vi "Place.vi"(4 "Side":T1=enum."right", 9 "Part Name":string="Large Gear", 11 "Location":T2={"x"=50.0, "y"=900.0, "a"=900.0, "Name"="Large Gear"}) -> (0 "error out":errorcluster)   [LabVIEW 2013]
uses:
  ROS/Code/SubVIs/BaxterSide.ctl
  Move/Move Reference.vi
  Move/Move XYZA.vi
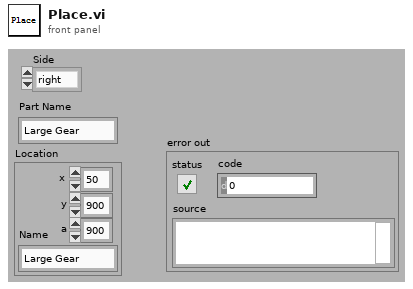
[diagram p1: front panel]
types:
  T1 = typedef "BaxterSide.ctl" = enum16{"left", "right"}
  T2 = cluster{"x":dbl, "y":dbl, "a":dbl, "Name":string}
  T3 = cluster{"X":dbl, "Y":dbl, "Z":dbl, "O":dbl, "A":dbl, "T":dbl}
  T4 = typedef "NI_Matrix.lvlib/RealMatrix.ctl" = dbl[][]
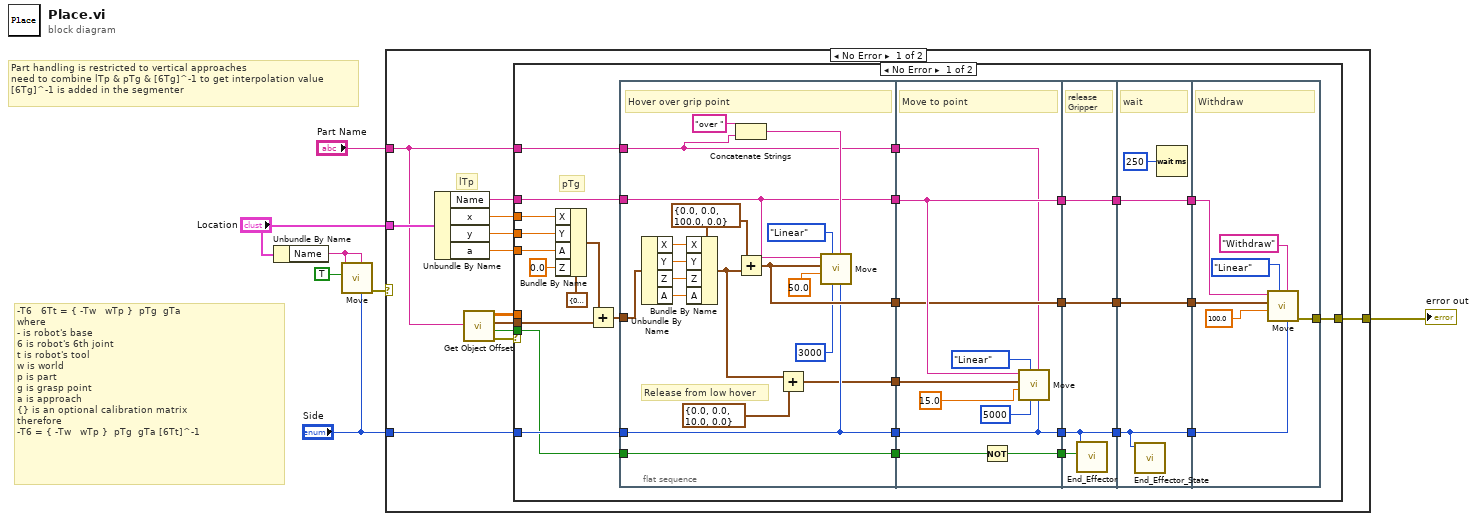
[diagram p0: block diagram]
diagram:
  # "Part handling is restricted to vertical approaches\nneed to combine lTp & pTg & [6Tg]^-1 to get interpolation value\n[6Tg]^-1 is added in the segmenter"
  # "-T6   6Tt = { -Tw   wTp }  pTg  gTa\nwhere \n- is robot's base\n6 is robot's 6th joint\nt is robot's tool\nw is world\np is part\ng is grasp point\na is approach\n{} is an optional calibration matrix\ntherefore\n-T6 = { -Tw   wTp }  pTg  gTa [6Tt]^-1"
  n1 = Unbundle By Name("Location") -> ("Name"=w3:string)
  n2 = call-poly "Move.vi"("Side"="Side", "Label"=w3, "To Reference"=TRUE, "Location"=w3) -> ("error out"=w5:errorcluster)  [unwired: 7 in]
  n3 = case shown="No Error" w5 {
    selector: w5 -> [_ w94]
    tunnel: [w19 w94] -> w7
    tunnel: "Location" -> [w13 _]
    tunnel: "Side" -> [w15 _]
    tunnel: "Part Name" -> [w8 _]
    frame No Error {
      # "lTp"
      n4 = Unbundle By Name(w13) -> ("Name"=w12:string, "x"=w11:dbl, "y"=w10:dbl, "a"=w9:dbl)
      n5 = call "Get Object Offset.vi"("Label"=w8) -> ("error out"=w17:errorcluster, "GraspClose"=w16:bool, "XYZOAT"=w14:T3, "T"=w18:T4)  [unwired: 7 in]
      n6 = case shown="No Error" w17 {
        selector: w17 -> [_ w93]
        tunnel: [w48 w93] -> w19
        tunnel: w18 -> [_ _]
        tunnel: w16 -> [w21 _]
        tunnel: w15 -> [w24 _]
        tunnel: w14 -> [w46 _]
        tunnel: w12 -> [w45 _]
        tunnel: w11 -> [w44 _]
        tunnel: w10 -> [w43 _]
        tunnel: w9 -> [w42 _]
        tunnel: w8 -> [w23 _]
        frame No Error {
          # "pTg"
          n7 = Bundle By Name(cluster=T3 {"X"=0.0, "Y"=0.0, "Z"=0.0, "O"=0.0, "A"=0.0, "T"=0.0} ("XYZOAT"), "X"=w44, "Y"=w43, "A"=w42, "Z"=0.0) -> (w47:T3)
          n8 = Add(x=w47, y=w46) -> (x+y=w40:T3)
          n9 = flat-sequence {
            tunnel: [w53] -> w39
            tunnel: [w55] -> w38
            tunnel: [w51] -> w37
            tunnel: [w57] -> w36
            tunnel: [w56] -> w35
            tunnel: w24 -> [w53]
            tunnel: w21 -> [w55]
            tunnel: w40 -> [w63]
            tunnel: w45 -> [w57]
            tunnel: w23 -> [w52]
            tunnel: [w52] -> w22
            tunnel: w39 -> [w71]
            tunnel: [w71] -> w34
            tunnel: w38 -> [w73]
            tunnel: [w68] -> w33
            tunnel: w37 -> [w75]
            tunnel: w36 -> [w74]
            tunnel: [w74] -> w32
            tunnel: w35 -> [w72]
            tunnel: [w72] -> w31
            tunnel: w22 -> [w69]
            tunnel: w34 -> [w79]
            tunnel: [w79] -> w30
            tunnel: w33 -> [w78]
            tunnel: w32 -> [w81]
            tunnel: [w81] -> w28
            tunnel: w31 -> [w80]
            tunnel: [w80] -> w26
            tunnel: w30 -> [w82]
            tunnel: [w82] -> w29
            tunnel: w28 -> [w85]
            tunnel: [w85] -> w27
            tunnel: w26 -> [w84]
            tunnel: [w84] -> w25
            tunnel: w29 -> [w86]
            tunnel: [w92] -> w48
            tunnel: w27 -> [w87]
            tunnel: w25 -> [w88]
            frame #0 {
              w58 = cluster{"X":dbl, "Y":dbl, "Z":dbl, "A":dbl} {"X"=0.0, "Y"=0.0, "Z"=100.0, "A"=0.0} ("XYZA")
              # "Release from low hover"
              # "Hover over grip point"
              n10 = Unbundle By Name(w63) -> ("X"=w62:dbl, "Y"=w61:dbl, "Z"=w60:dbl, "A"=w59:dbl)
              n11 = Bundle By Name(cluster=w58, "X"=w62, "Y"=w61, "Z"=w60, "A"=w59) -> (w49:cluster{"X":dbl, "Y":dbl, "Z":dbl, "A":dbl})
              n12 = Concatenate Strings("over " ("string"), w52) -> (w64:string)
              n13 = Add(x=w58, y=w49) -> (x+y=w56:cluster{"X":dbl, "Y":dbl, "Z":dbl, "A":dbl})
              n14 = Add(x=w49, y=cluster{"X":dbl, "Y":dbl, "Z":dbl, "A":dbl} {"X"=0.0, "Y"=0.0, "Z"=10.0, "A"=0.0} ("XYZA")) -> (x+y=w51:cluster{"X":dbl, "Y":dbl, "Z":dbl, "A":dbl})
              n15 = call-poly "Move.vi"("Side"=w53, "Label"=w64, "Wait Time"=3000, "Motion"=enum16{"Joint", "Linear"}."Linear", "Speed (mm/s)"=50.0, "XYZA"=w56, "Location"=w57) -> ()  [unwired: 4 in, 1 out]
            }
            frame #1 {
              # "Move to point"
              n16 = Not(x=w73) -> (.not. x?=w68:bool)
              n17 = call-poly "Move.vi"("Side"=w71, "Label"=w69, "Wait Time"=5000 ("milliseconds to wait"), "Motion"=enum16{"Joint", "Linear"}."Linear", "Speed (mm/s)"=15.0, "XYZA"=w75, "Location"=w74) -> ()  [unwired: 4 in, 1 out]
            }
            frame #2 {
              # "release Gripper"
              n18 = call "End_Effector.vi"("Close"=w78, "Side"=w79) -> ()  [unwired: 6 in, 1 out]
            }
            frame #3 {
              # "wait"
              n19 = call "End_Effector_State.vi"("Side"=w82) -> ()  [unwired: 5 in, 3 out]
              n20 = Wait (ms)(milliseconds to wait=u32 250) -> ()  [unwired: 1 out]
            }
            frame #4 {
              # "Withdraw"
              n21 = call-poly "Move.vi"("Side"=w86, "Label"="Withdraw", "Motion"=enum16{"Joint", "Linear"}."Linear", "Speed (mm/s)"=100.0, "XYZA"=w88, "Location"=w87) -> ("error out"=w92:errorcluster)  [unwired: 5 in]
            }
          }
        }
        frame Error {
        }
      }
    }
    frame Error {
    }
  }
  "error out" <- w7
